vi "Trigger.vi"(8 "error in (no error)":errorcluster, 11 "Process Controller in":refnum<class "Process Controller.lvclass">) -> (0 "error out":errorcluster, 3 "Process Controller out":refnum<class "Process Controller.lvclass">)   [LabVIEW 2019, in "Process Controller.lvclass"]
uses:
  Process Controller.lvclass
  C:/GitHub/LabActor/Worker/Worker.lvclass
  Worker/Worker.lvclass/Worker.ctl
  Process Controller.lvclass/Process Controller.ctl
  <vilib>/ActorFramework/Message Enqueuer/Message Enqueuer.lvclass/Message Enqueuer.ctl
  Template Module/Read State.vi
  Read Active measurements enqueuers.vi
  <vilib>/ActorFramework/Message Enqueuer/Enqueue.vi
  Worker Messages/Trigger Msg/Trigger Msg.lvclass
  C:/Program Files/National Instruments/LabVIEW 2019/vi.lib/ActorFramework/Message/Message.lvclass
  <vilib>/ActorFramework/Message Priority Queue/Priority Enqueue.vi
  <vilib>/ActorFramework/Message Enqueuer/Message Enqueuer.lvclass
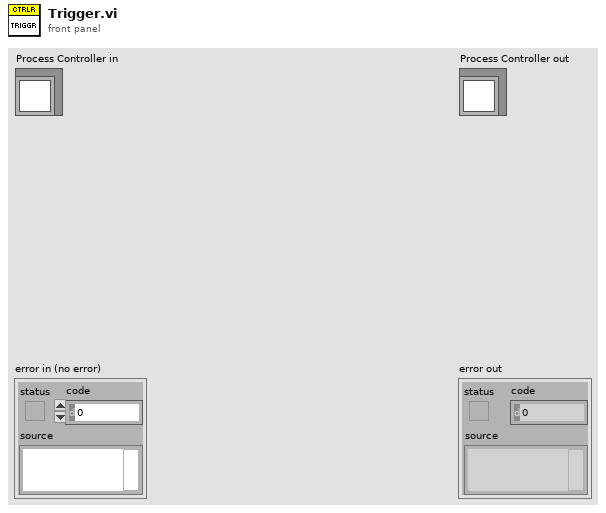
[diagram p1: front panel]
types:
  T1 = typedef "Worker State.ctl" = enum16{"Idle", "Starting", "Working", "Stopping"}
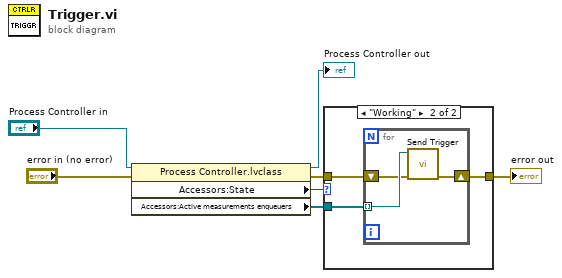
[diagram p0: block diagram]
diagram:
  n1 = property class="Process Controller.lvclass"(reference="Process Controller in", error in="error in (no error)") -> (reference out=→"Process Controller out":refnum<class "Process Controller.lvclass">, error out=w3:errorcluster, "Accessors:State"=w6:T1, "Accessors:Active measurements enqueuers"=w5:refnum<class "Message Enqueuer.lvclass">[])
  n2 = case shown="\"Working\"" w6 {
    tunnel: w5 -> [_ w11]
    tunnel: w3 -> [w8 w10]
    tunnel: [w8 w9] -> w2
    frame "Idle", Default {
    }
    frame "Working" {
      n3 = for {
        tunnel: w11 -> [w14] mode=indexing
        shift-right: [w12] -> w9
        shift-left: w10 -> [w13]
        n4 = call "Send Trigger.vi"("error in (no error)"=w13, "Message Enqueuer"=w14) -> ("error out"=w12:errorcluster)  [unwired: 8 in, 1 out]
      }
    }
  }
  "error out" <- w2
